vi "Run 0mqComm.vi"(8 "error in (no error)":errorcluster, 9 "show FP":bool, 10 "channel configuration":T1, 11 "Messenger in":refnum<class "Messenger.lvclass">) -> (0 "error out":errorcluster, 3 "Messenger out":refnum<class "Messenger.lvclass">)   [LabVIEW 2018, in "Messenger.lvclass"]
uses:
  Messenger.lvclass
  Messenger.lvclass/Messenger.ctl
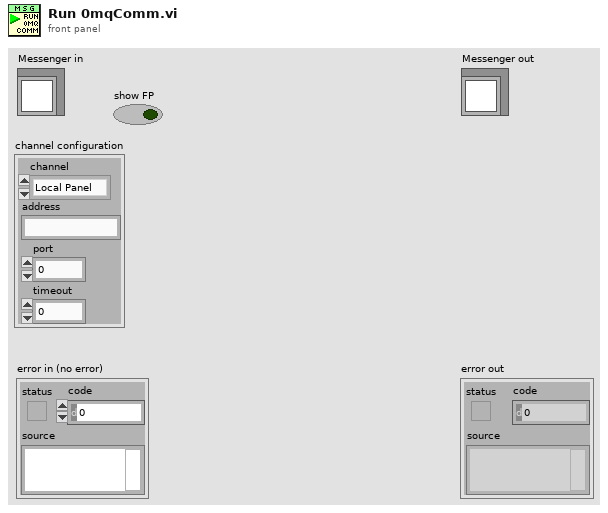
[diagram p1: front panel]
types:
  T1 = cluster{"channel":enum32{"Local Panel", "Inner TCP/IP", "Outer TCP/IP", "MQTT", "ZeroMQ"}, "address":string, "port":u16, "timeout":i32}
  T2 = cluster{"S4commandQueueName":string, "S4statusQueueName":string, "comm configuration":cluster{"channel":enum32{"Local Panel", "Inner TCP/IP", "Outer TCP/IP", "MQTT", "ZeroMQ"}, "address":string, "port":u16, "timeout":i32}}
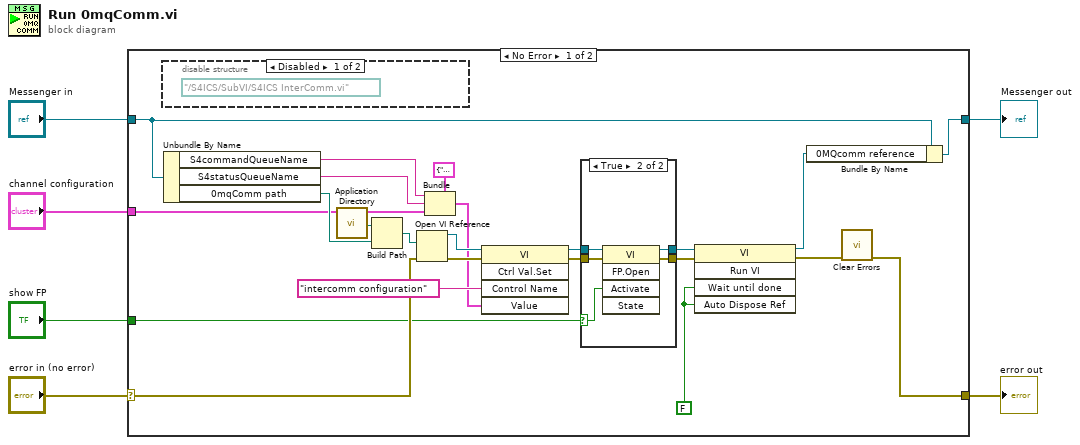
[diagram p0: block diagram]
diagram:
  n1 = case shown="No Error" "error in (no error)" {
    selector: "error in (no error)" -> [w21 w37]
    tunnel: [w20 w37] -> w5
    tunnel: [w29 w38] -> w3
    tunnel: "Messenger in" -> [w16 w38]
    tunnel: "show FP" -> [w18 _]
    tunnel: "channel configuration" -> [w8 _]
    frame No Error {
      w23 = FALSE
      n2 = disable-structure shown="Disabled" {
        frame Disabled {
          (unwired) path "../S4ICS/SubVI/S4ICS InterComm.vi" ("name or relative path")
        }
        frame Enabled {
        }
      }
      n3 = Unbundle By Name(w16) -> ("S4commandQueueName"=w12:string, "S4statusQueueName"=w11:string, "0mqComm path"=w9:path)
      n4 = call <vilib>:"Application Directory.vi"() -> ("Application Directory"=w17:path)
      n5 = Build Path(base path=w17, name or relative path=w9) -> (appended path=w28:path)
      n6 = Open VI Reference(vi path=w28, error in (no error)=w21) -> (vi reference=w26:refnum<vi>, error out=w27:errorcluster)  [unwired: 4 in]
      n7 = Bundle(cluster=T2 {"S4commandQueueName"="", "S4statusQueueName"="", "comm configuration"={"channel"=enum."Local Panel", "address"="", "port"=0, "timeout"=0}} ("intercomm configuration"), "S4commandQueueName"=w12, "S4statusQueueName"=w11, "comm configuration"=w8) -> (w10:T2)
      n8 = invoke class="VI" method="Ctrl Val.Set"(reference=w26, error in=w27, "Control Name"="intercomm configuration", "Value"=w10) -> (reference out=w14:refnum<vi>, error out=w15:errorcluster)  [unwired: 1 in, 3 out]
      n9 = case shown="True" w18 {
        selector: w18 -> [_ w34]
        tunnel: [w31 w36] -> w25
        tunnel: w14 -> [w31 w35]
        tunnel: w15 -> [w30 w33]
        tunnel: [w30 w32] -> w24
        frame False {
        }
        frame True {
          n10 = invoke class="VI" method="FP.Open"(reference=w35, error in=w33, "Activate"=w34) -> (reference out=w36:refnum<vi>, error out=w32:errorcluster)  [unwired: 2 in, 3 out]
        }
      }
      n11 = invoke class="VI" method="Run VI"(reference=w25, error in=w24, "Wait until done"=w23, "Auto Dispose Ref"=w23) -> (reference out=w19:refnum<vi>, error out=w22:errorcluster)  [unwired: 1 in, 3 out]
      n12 = Bundle By Name(cluster=w16, "0MQcomm reference"=w19) -> (w29:refnum<class "Messenger.lvclass">)
      n13 = call <vilib>:"Clear Errors.vi"("error in (no error)"=w22) -> ("error out"=w20:errorcluster)  [unwired: 5 in, 1 out]
    }
    frame Error {
    }
  }
  "error out" <- w5
  "Messenger out" <- w3
